vi "Create all RT FIFOS.vi"(8 "error in":errorcluster) -> (0 "error out":errorcluster, 3 "RT FIFOs--cluster":T1)   [LabVIEW 2021, in "RT Main.lvlib"]
uses:
  RT Main.lvlib
  RT FIFOS--cluster.ctl
  Libraries/Common RT/Hardware Monitoring.ctl
  Libraries/Common RT/Common RT.lvlib
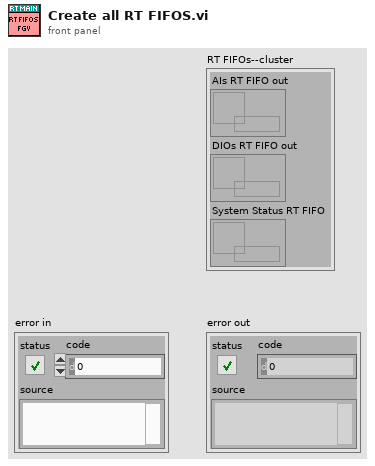
[diagram p1: front panel]
types:
  T1 = typedef "RT Main.lvlib/RT FIFOS--cluster.ctl" = cluster{"AIs RT FIFO out":refnum<k33>, "DIOs RT FIFO out":refnum<k33>, "System Status RT FIFO":refnum<k33>}
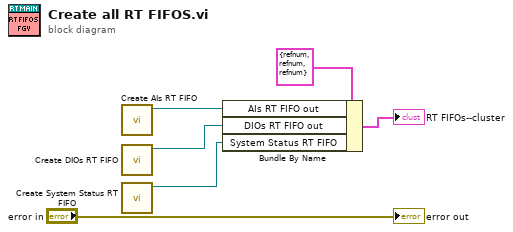
[diagram p0: block diagram]
diagram:
  n1 = call "Create AIs RT FIFO.vi"() -> ("AIs RT FIFO out"=w5:refnum<k33>)  [unwired: 10 in, 1 out]
  n2 = call "Create DIOs RT FIFO.vi"() -> ("DIOs RT FIFO out"=w4:refnum<k33>)  [unwired: 10 in, 1 out]
  n3 = call "Create System Status RT FIFO.vi"() -> ("System Status RT FIFO"=w1:refnum<k33>)  [unwired: 10 in, 1 out]
  n4 = Bundle By Name(cluster=T1 {"AIs RT FIFO out"=refnum, "DIOs RT FIFO out"=refnum, "System Status RT FIFO"=refnum}, "AIs RT FIFO out"=w5, "DIOs RT FIFO out"=w4, "System Status RT FIFO"=w1) -> (→"RT FIFOs--cluster":T1)
  "error out" <- "error in"
